vi "Copy Image (Greyscale).vi"(8 "error in (no error)":errorcluster, 10 "Greyscale Image Destination":T1, 11 "Greyscale Image Source":T1) -> (0 "error out":errorcluster, 3 "Greyscale Image Destination (duplicate)":T1)   [LabVIEW 2020, in "g_ar_toolkit.image.lvlib"]
uses:
  g_ar_toolkit.image.lvlib
  Greyscale Image.ctl
  c92252ab-1097-45af-a449-7a3c8cf05290.vi
  g_ar_toolkit.common/Module Path.vi
  <vilib>/Utility/error.llb/Error Cluster From Error Code.vi
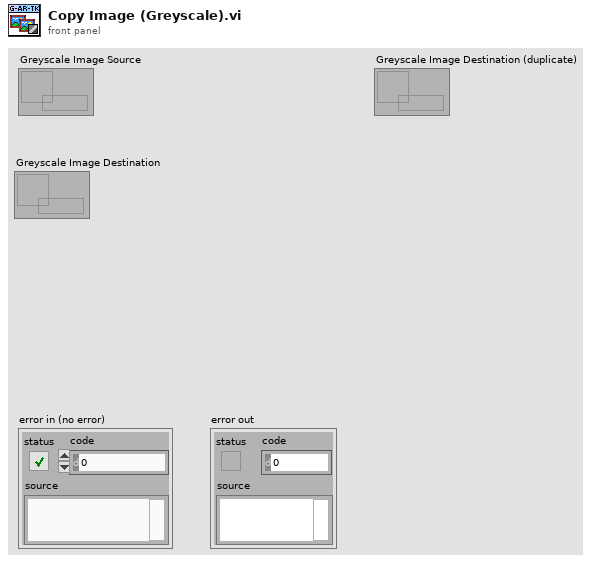
[diagram p1: front panel]
types:
  T1 = typedef "g_ar_toolkit.image.lvlib/Greyscale Image.ctl" = refnum<data-value>
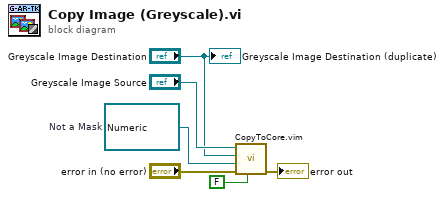
[diagram p0: block diagram]
diagram:
  w1 = refnum<data-value> refnum  # Not a Mask
  n1 = call "CopyToCore.vim"("Has Mask"=FALSE, "error in (no error)"="error in (no error)", "Mask"=w1, "Dst"="Greyscale Image Destination", "Src"="Greyscale Image Source") -> ("error out"=→"error out":errorcluster)  [unwired: 6 in]
  "Greyscale Image Destination (duplicate)" <- "Greyscale Image Destination"
